vi "Bloomy BS120x Data Logging Example.vi"() -> ()   [LabVIEW 2021]
uses:
  src/TypeDefs/UnitType.ctl
  src/Public/New BS120x Device/New BS120x Ethernet Device.vi
  src/Public/New BS120x Device/New BS120x XNET Device.vi
  src/BS120x.lvclass
  src/BS120x Driver.lvlib
panel:
  in  "Tab Control":enum32{"Basic Control", "Plotting"}(tab)
  out "Protocol":enum32{"CAN", "Ethernet"}(tab)=enum."Ethernet"
  out "Box IDs":u8[](array[numeric])=[1]
  in  "CAN Interface":refnum<k21>
  in  "Current Box ID":u8
  out "Box IP address":string="192.168.1.101"
  out "TCP port":u16=12345
  out "UDP port":u16=54321
  in  "Reset Unit":bool
  in  "Voltage":dbl=5.0 min=0.0 max=5.0 step=0.5
  in  "Source \nCurrent":dbl
  in  "Sink \nCurrent":dbl
  in  "State":bool
  out "Cell Voltages":dbl[](array[numeric])
  out "Cell Current":dbl[](array[numeric]) format="%#8.1f"
  in  "PID Disable":bool
  in  "Precision":bool
  out "Unit Type":T1=enum."BS1201"
  in  "Channel":u16(ring) items=["All", "1", "2", "3", "4", "5", "6", "7", "8", "9", "10", "11", "12"]
  out "error out":errorcluster
  in  "Logging State":enum32{"On", "Off"}(radio)
  in  "Data Log Path":path
  out "Cell Voltages":T2(graph)
  out "Cell Currents":T3(graph)
  in  "Acquisition Rate (Hz)":i32=100 min=1 max=100 step=1
  in  "stop":bool
  # "(c) 2025 Bloomy Controls, Inc. All rights reserved."
  # "Initialization & Configuration"
  # "Cell Control & Readback"
  # "Readback Data"
  # "Control Outputs"
  # "1"
  # "V"
  # "6"
  # "mA"
  # "Operational Config\n(BS1201 Only)"
  # "mA"
  # "12"
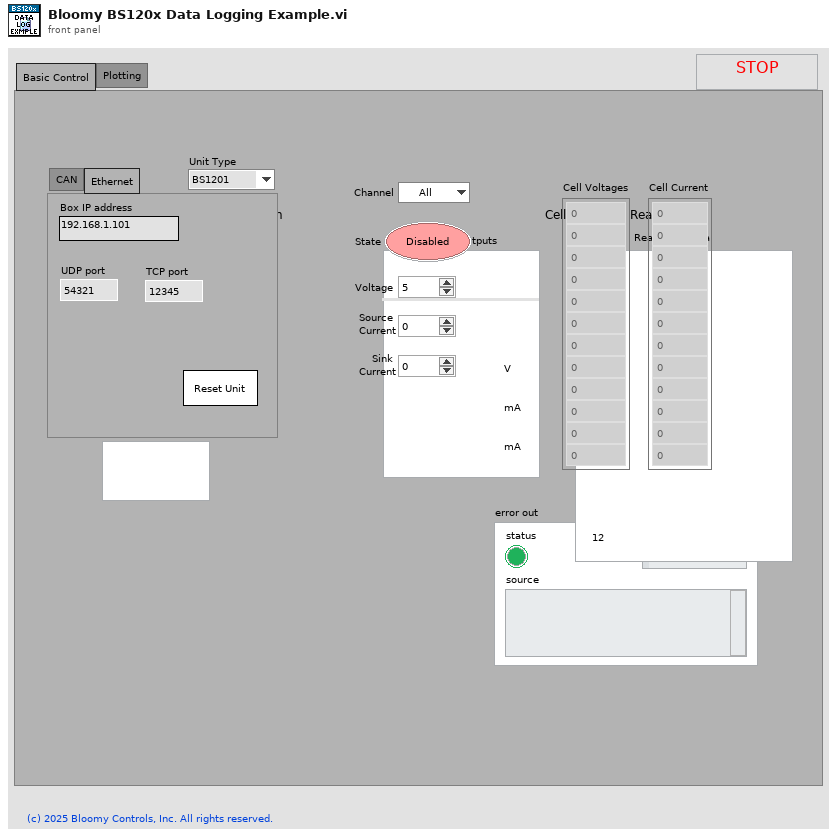
[diagram p1: front panel]
types:
  T1 = typedef "BS120x Driver.lvlib/BS120x.lvclass/UnitType.ctl" = enum16{"BS1200", "BS1201"}
  T2 = cluster{"Voltage[0]":dbl, "Voltage[1]":dbl, "Voltage[2]":dbl, "Voltage[3]":dbl, "Voltage[4]":dbl, "Voltage[5]":dbl, "Voltage[6]":dbl, "Voltage[7]":dbl, "Voltage[8]":dbl, "Voltage[9]":dbl, "Voltage[10]":dbl, "Voltage[11]":dbl}
  T3 = cluster{"Current[0]":dbl, "Current[1]":dbl, "Current[2]":dbl, "Current[3]":dbl, "Current[4]":dbl, "Current[5]":dbl, "Current[6]":dbl, "Current[7]":dbl, "Current[8]":dbl, "Current[9]":dbl, "Current[10]":dbl, "Current[11]":dbl}
  T4 = typedef "BS120x Driver.lvlib/DiscoveredDevice.ctl" = cluster{"Unit Type":T1, "Serial Number":string, "Protocol":T5, "IP Address":string, "UDP Port":u16, "TCP Port":u16, "XNET Box ID":u8, "OS":string, "Firmware Version":string}
  T5 = typedef "BS120x Driver.lvlib/BS120x.lvclass/Protocol.ctl" = enum16{"CAN", "Ethernet"}
  T6 = enum16{"open", "replace", "create", "open or create", "replace or create", "replace or create with confirmation"}
  T7 = cluster{"name (unnamed)":string, "name (unnamed)":string}
  T8 = cluster{"name (unnamed)":string, "NewVal":enum32{"On", "Off"}}
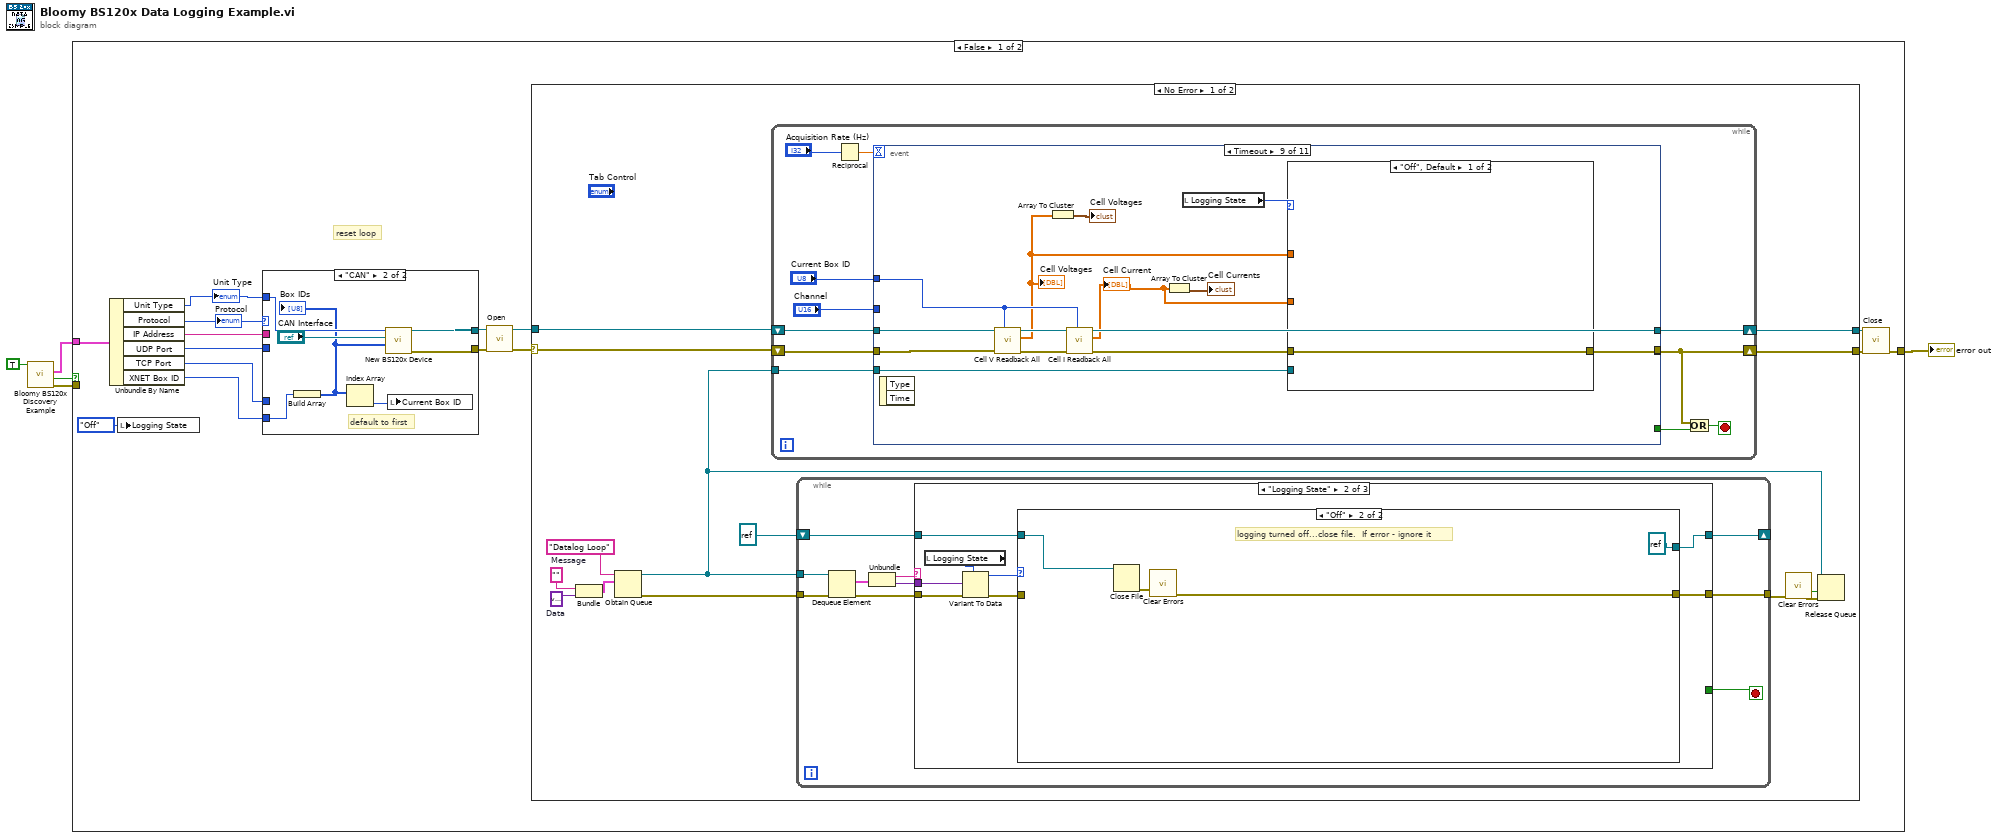
[diagram p0: block diagram]
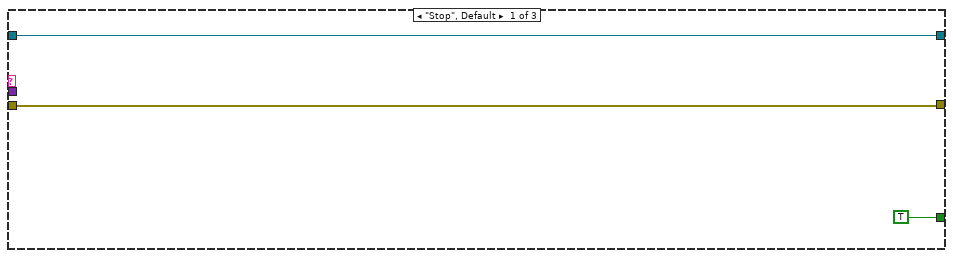
[diagram p2: hidden frame]
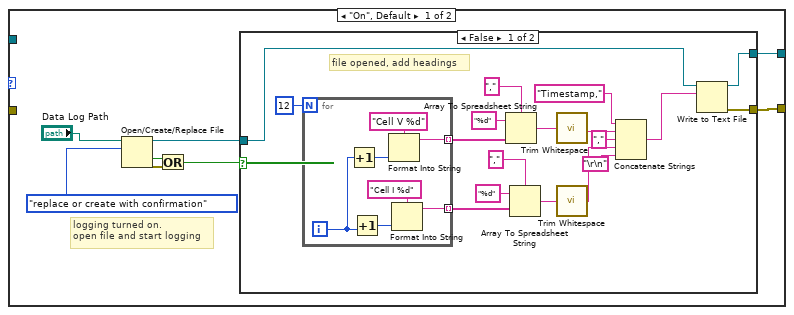
[diagram p3: hidden frame]
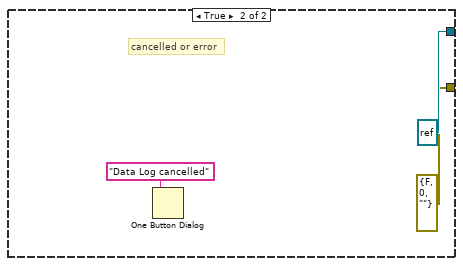
[diagram p4: hidden frame]
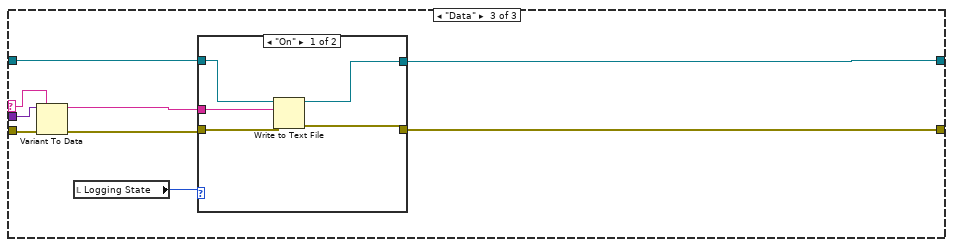
[diagram p5: hidden frame]
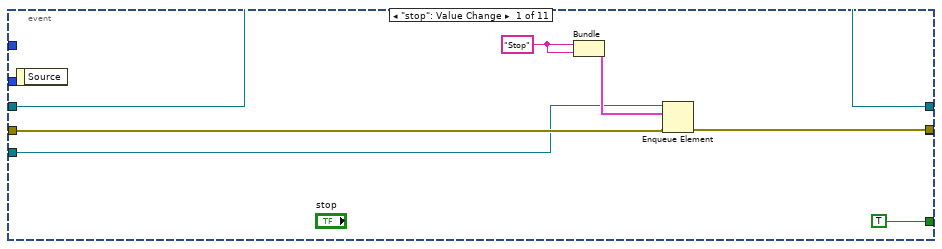
[diagram p7: hidden frame]
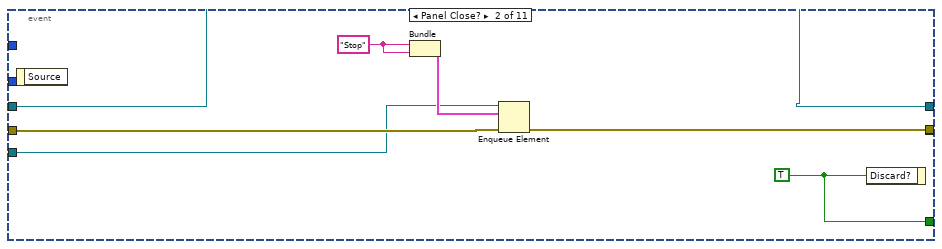
[diagram p8: hidden frame]
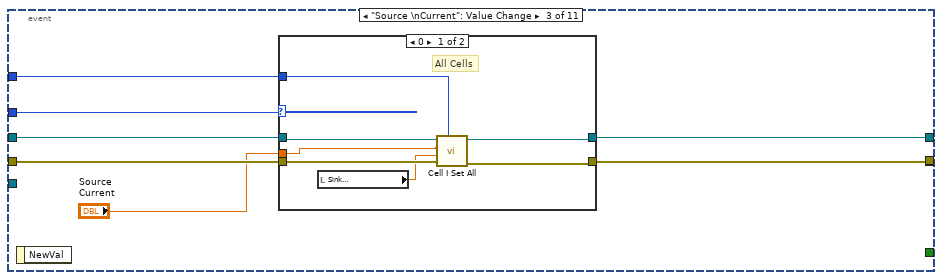
[diagram p9: hidden frame]
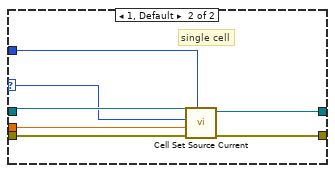
[diagram p10: hidden frame]
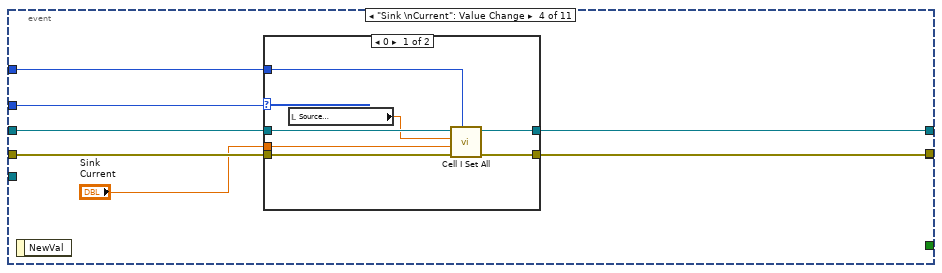
[diagram p11: hidden frame]
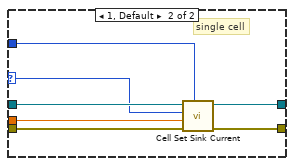
[diagram p12: hidden frame]
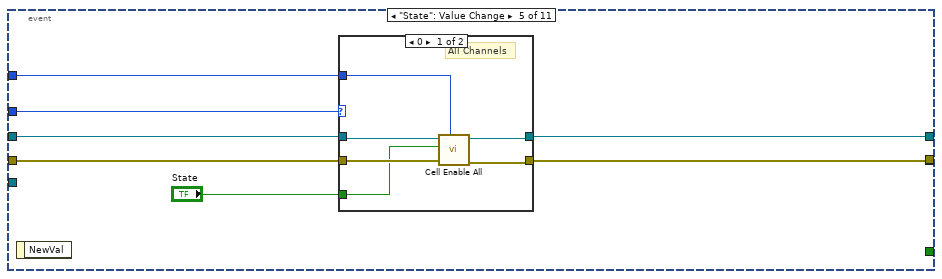
[diagram p13: hidden frame]
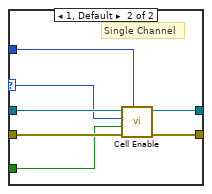
[diagram p14: hidden frame]
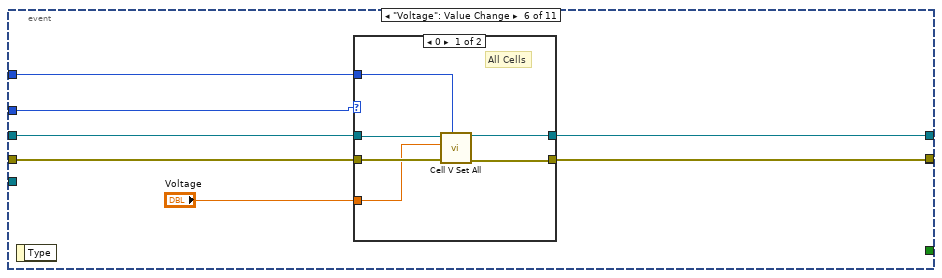
[diagram p15: hidden frame]
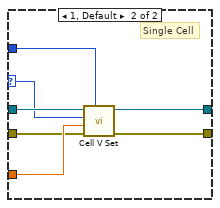
[diagram p16: hidden frame]
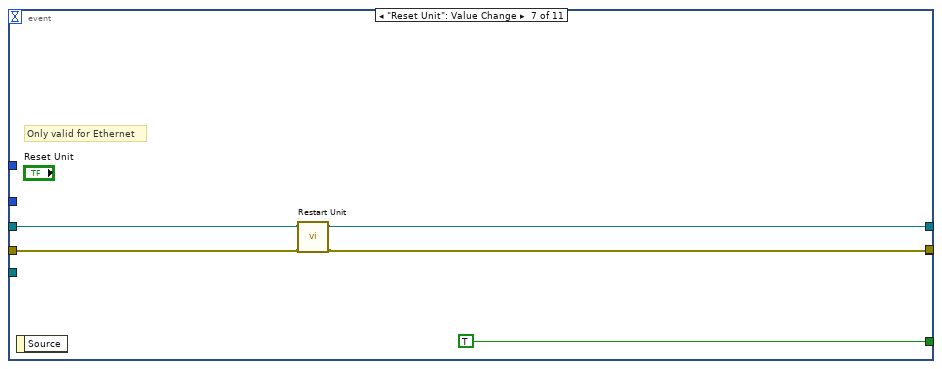
[diagram p17: hidden frame]
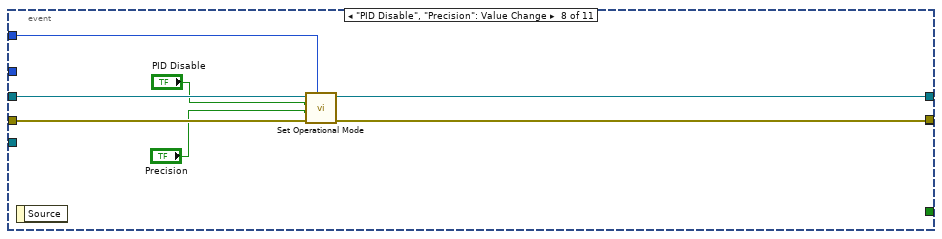
[diagram p18: hidden frame]
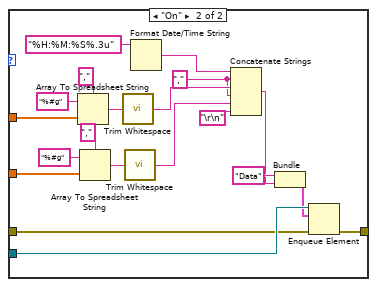
[diagram p19: hidden frame]
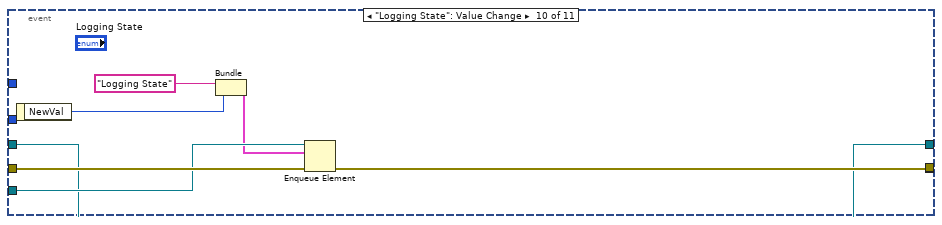
[diagram p20: hidden frame]
diagram:
  n1 = call "Bloomy BS120x Discovery Example.vi"("Allow Selection"=TRUE) -> ("error out"=w2:errorcluster, "Canceled"=w3:bool, "Selected Device"=w1:T4)  [unwired: 7 in, 1 out]
  n2 = case shown="False" w3 {
    tunnel: [w15 w290] -> w5
    tunnel: w2 -> [_ w290]
    tunnel: w1 -> [w13 _]
    frame False {
      # "reset loop"
      n3 = Unbundle By Name(w13) -> ("Unit Type"=w12:T1, "Protocol"=w11:T5, "IP Address"=w10:string, "UDP Port"=w9:u16, "TCP Port"=w8:u16, "XNET Box ID"=w7:u8)
      "Unit Type" <- w12
      "Protocol" <- w11
      n4 = local write "Logging State"(enum32{"On", "Off"}."Off" ("Logging State")) -> ()
      n5 = case shown="\"CAN\"" w11 {
        tunnel: w12 -> [w282 w287]
        tunnel: [w281 w289] -> w18
        tunnel: [w280 w288] -> w16
        tunnel: w10 -> [w279 _]
        tunnel: w9 -> [w278 _]
        tunnel: w8 -> [w277 _]
        tunnel: w7 -> [_ w283]
        frame "Ethernet", Default {
          n6 = call-poly "New BS120x Device.vi"("TCP port"=w277, "UDP port"=w278, "Box IP address"=w279, "Unit Type"=w282) -> ("error out"=w280:errorcluster, "BS120x Out"=w281:refnum<class "BS120x.lvclass">)  [unwired: 6 in]
          "Box IP address" <- w279
          "TCP port" <- w277
          "UDP port" <- w278
        }
        frame "CAN" {
          # "default to first"
          n7 = Build Array(w283) -> (w284:u8[])
          "Box IDs" <- w284
          n8 = Index Array(array=w284) -> (element=w285:u8)  [unwired: 1 in]
          n9 = call-poly "New BS120x Device.vi"("Box IDs"=w284, "CAN Interface"="CAN Interface", "Unit Type"=w287) -> ("error out"=w288:errorcluster, "BS120x out"=w289:refnum<class "BS120x.lvclass">)  [unwired: 7 in]
          n10 = local write "Current Box ID"(w285) -> ()
        }
      }
      n11 = call-dynamic "Open.vi"("error in (no error)"=w16, "BS120x in"=w18) -> ("error out"=w14:errorcluster, "BS120x out"=w17:refnum<class "BS120x.lvclass">)  [unwired: 8 in]
      n12 = case shown="No Error" w14 {
        selector: w14 -> [w31 w275]
        tunnel: [w34 w275] -> w20
        tunnel: [w33 w276] -> w19
        tunnel: w17 -> [w32 w276]
        frame No Error {
          w27 = variant  # Data
          w28 = ""  # Message
          n13 = Bundle("Message"=w28, "Data"=w27) -> (w26:cluster{"Message":string, "Data":variant})  [unwired: 1 in]
          n14 = Obtain Queue(name (unnamed)="Datalog Loop", element data type=w26) -> (queue out=w21:refnum<queue>, error out=w25:errorcluster)  [unwired: 3 in, 1 out]
          n15 = while {
            shift-right: [w117] -> w34
            shift-left: w31 -> [w120]
            shift-right: [w122] -> w33
            shift-left: w32 -> [w121]
            tunnel: w21 -> [w112]
            stop <- w119 stop-if-true
            n16 = Reciprocal(x="Acquisition Rate (Hz)") -> (1/x=w113:dbl)
            n17 = event shown="[8] Timeout" {
              selector: _ -> [_ _ _ _ _ _ _ _ _ _ _]
              dyn-events: _ -> [_ _ _ _ _ _ _ _ _ _ _]
              timeout: w113 -> [_ _ _ _ _ _ _ _ _ _ _]
              tunnel: [w128 w133 w140 w161 w183 w201 w220 w227 w244 w267 w274] -> w122
              tunnel: w121 -> [w128 w133 w143 w164 w184 w204 w219 w228 w232 w267 w274]
              tunnel: [w126 _ w141 w160 w182 w202 w221 w229 w239 w268 w273] -> w117
              tunnel: w120 -> [w127 w132 w142 w163 w185 w203 w222 w230 w231 w272 w273]
              tunnel: [TRUE ("Discard?") w136 _ _ _ _ TRUE ("Discard?") _ _ _ _] -> w118
              tunnel: "Channel" -> [_ _ w138 w159 w180 w200 _ _ _ _ _]
              tunnel: "Current Box ID" -> [_ _ w137 w158 w179 w199 _ w224 w241 _ _]
              tunnel: w112 -> [w125 w130 _ _ _ _ _ _ w233 w271 _]
              tunnel: [_ w131 _ _ _ _ _ _ _ _ _] -> _
              event "stop": Value Change {
                w124 = "Stop" ("name (unnamed)")
                n18 = event-data() -> ()  [unwired: 1 in, 1 out]
                n19 = Bundle("name (unnamed)"=w124, "name (unnamed)"=w124) -> (w129:T7)  [unwired: 1 in]
                n20 = Enqueue Element(queue=w125, element=w129, error in (no error)=w127) -> (error out=w126:errorcluster)  [unwired: 1 in, 2 out]
              }
              event Panel Close? {
                w134 = "Stop" ("name (unnamed)")
                w136 = TRUE ("Discard?")
                n21 = event-data() -> ()  [unwired: 1 in, 1 out]
                n22 = Bundle("name (unnamed)"=w134, "name (unnamed)"=w134) -> (w135:T7)  [unwired: 1 in]
                n23 = Enqueue Element(queue=w130, element=w135, error in (no error)=w132) -> (error out=w131:errorcluster)  [unwired: 1 in, 2 out]
                n24 = event-data("Discard?"=w136) -> ()  [unwired: 1 in, 1 out]
              }
              event "Source \nCurrent": Value Change {
                n25 = event-data() -> ()  [unwired: 1 in, 1 out]
                n26 = case shown="0" w138 {
                  selector: w138 -> [_ w152]
                  tunnel: w143 -> [w149 w157]
                  tunnel: w142 -> [w148 w156]
                  tunnel: [w147 w155] -> w141
                  tunnel: [w150 w154] -> w140
                  tunnel: "Source \nCurrent" -> [w146 w153]
                  tunnel: w137 -> [w144 w151]
                  frame 0 {
                    # "All Cells"
                    n27 = local read "Sink \nCurrent"() -> (w145:dbl)
                    n28 = call-dynamic "Cell I Set All.vi"("Box ID"=w144, "error in (no error)"=w148, "Sink I All"=w145, "Source I All"=w146, "BS120x in"=w149) -> ("error out"=w147:errorcluster, "BS120x out"=w150:refnum<class "BS120x.lvclass">)  [unwired: 5 in]
                  }
                  frame 1, Default {
                    # "single cell"
                    n29 = call-dynamic "Cell Set Source Current.vi"("Box ID"=w151, "error in (no error)"=w156, "Source Current Limit (mA)"=w153, "Channel"=w152, "BS120x in"=w157) -> ("error out"=w155:errorcluster, "BS120x out"=w154:refnum<class "BS120x.lvclass">)  [unwired: 5 in]
                  }
                }
              }
              event "Sink \nCurrent": Value Change {
                n30 = event-data() -> ()  [unwired: 1 in, 1 out]
                n31 = case shown="0" w159 {
                  selector: w159 -> [_ w173]
                  tunnel: w164 -> [w169 w178]
                  tunnel: w163 -> [w168 w177]
                  tunnel: "Sink \nCurrent" -> [w167 w176]
                  tunnel: [w170 w175] -> w161
                  tunnel: [w171 w174] -> w160
                  tunnel: w158 -> [w165 w172]
                  frame 0 {
                    n32 = local read "Source \nCurrent"() -> (w166:dbl)
                    n33 = call-dynamic "Cell I Set All.vi"("Box ID"=w165, "error in (no error)"=w168, "Sink I All"=w167, "Source I All"=w166, "BS120x in"=w169) -> ("error out"=w171:errorcluster, "BS120x out"=w170:refnum<class "BS120x.lvclass">)  [unwired: 5 in]
                  }
                  frame 1, Default {
                    # "single cell"
                    n34 = call-dynamic "Cell Set Sink Current.vi"("Box ID"=w172, "error in (no error)"=w177, "Sink Current Limit (mA)"=w176, "Channel"=w173, "BS120x in"=w178) -> ("error out"=w174:errorcluster, "BS120x out"=w175:refnum<class "BS120x.lvclass">)  [unwired: 5 in]
                  }
                }
              }
              event "State": Value Change {
                n35 = event-data() -> ()  [unwired: 1 in, 1 out]
                n36 = case shown="0" w180 {
                  selector: w180 -> [_ w193]
                  tunnel: w185 -> [w190 w198]
                  tunnel: w184 -> [w191 w197]
                  tunnel: [w189 w196] -> w183
                  tunnel: [w188 w195] -> w182
                  tunnel: "State" -> [w187 w194]
                  tunnel: w179 -> [w186 w192]
                  frame 0 {
                    # "All Channels"
                    n37 = call-dynamic "Cell Enable All.vi"("Box ID"=w186, "error in (no error)"=w190, "Enable"=w187, "BS120x in"=w191) -> ("error out"=w188:errorcluster, "BS120x out"=w189:refnum<class "BS120x.lvclass">)  [unwired: 6 in]
                  }
                  frame 1, Default {
                    # "Single Channel"
                    n38 = call-dynamic "Cell Enable.vi"("Box ID"=w192, "error in (no error)"=w198, "Enable"=w194, "Channel"=w193, "BS120x in"=w197) -> ("error out"=w195:errorcluster, "BS120x out"=w196:refnum<class "BS120x.lvclass">)  [unwired: 5 in]
                  }
                }
              }
              event "Voltage": Value Change {
                n39 = event-data() -> ()  [unwired: 1 in, 1 out]
                n40 = case shown="0" w200 {
                  selector: w200 -> [_ w213]
                  tunnel: "Voltage" -> [w207 w218]
                  tunnel: w204 -> [w211 w217]
                  tunnel: w203 -> [w210 w216]
                  tunnel: [w209 w215] -> w202
                  tunnel: [w208 w214] -> w201
                  tunnel: w199 -> [w206 w212]
                  frame 0 {
                    # "All Cells"
                    n41 = call-dynamic "Cell V Set All.vi"("Box ID"=w206, "error in (no error)"=w210, "Voltage"=w207, "BS120x in"=w211) -> ("error out"=w209:errorcluster, "BS120x out"=w208:refnum<class "BS120x.lvclass">)  [unwired: 6 in]
                  }
                  frame 1, Default {
                    # "Single Cell"
                    n42 = call-dynamic "Cell V Set.vi"("Box ID"=w212, "error in (no error)"=w216, "Voltage"=w218, "Channel"=w213, "BS120x in"=w217) -> ("error out"=w215:errorcluster, "BS120x out"=w214:refnum<class "BS120x.lvclass">)  [unwired: 5 in]
                  }
                }
              }
              event "Reset Unit": Value Change {
                # "Only valid for Ethernet"
                n43 = event-data() -> ()  [unwired: 1 in, 1 out]
                n44 = call-dynamic "Restart Unit.vi"("error in (no error)"=w222, "BS120x in"=w219) -> ("error out"=w221:errorcluster, "BS120x out"=w220:refnum<class "BS120x.lvclass">)  [unwired: 8 in]
              }
              event "PID Disable", "Precision": Value Change {
                n45 = event-data() -> ()  [unwired: 1 in, 1 out]
                n46 = call-dynamic "Set Operational Mode.vi"("Box ID"=w224, "error in (no error)"=w230, "Precision Mode"="Precision", "PID Disable"="PID Disable", "BS120x in"=w228) -> ("error out"=w229:errorcluster, "BS120x out"=w227:refnum<class "BS120x.lvclass">)  [unwired: 5 in]
              }
              event Timeout {
                n47 = event-data() -> ()  [unwired: 1 in, 2 out]
                n48 = call-dynamic "Cell V Readback All.vi"("Box ID"=w241, "error in (no error)"=w231, "BS120x in"=w232) -> ("error out"=w242:errorcluster, "Voltage"=w234:dbl[], "BS120x out"=w243:refnum<class "BS120x.lvclass">)  [unwired: 6 in]
                "Cell Voltages" <- w234
                n49 = Array To Cluster(array=w234) -> (cluster=→"Cell Voltages":T2)
                n50 = call-dynamic "Cell I Readback All.vi"("Box ID"=w241, "error in (no error)"=w242, "BS120x in"=w243) -> ("error out"=w240:errorcluster, "Current"=w235:dbl[], "BS120x out"=w244:refnum<class "BS120x.lvclass">)  [unwired: 6 in]
                "Cell Current" <- w235
                n51 = Array To Cluster(array=w235) -> (cluster=→"Cell Currents":T3)
                n52 = local read "Logging State"() -> (w238:enum32{"On", "Off"})
                n53 = case shown="\"Off\", Default" w238 {
                  tunnel: w234 -> [_ w265]
                  tunnel: w235 -> [_ w258]
                  tunnel: w240 -> [w245 w246]
                  tunnel: [w245 w251] -> w239
                  tunnel: w233 -> [_ w250]
                  frame "Off", Default {
                  }
                  frame "On" {
                    w252 = "," ("string")
                    n54 = Array To Spreadsheet String(delimiter (Tab)=",", array=w265, 3:"%#g" ("format string")) -> (spreadsheet string=w262:string)
                    n55 = Array To Spreadsheet String(delimiter (Tab)=",", array=w258, 3:"%#g" ("format string")) -> (spreadsheet string=w261:string)
                    n56 = call <vilib>:"Trim Whitespace.vi"("string"=w262) -> ("trimmed string"=w257:string)  [unwired: 1 in]
                    n57 = call <vilib>:"Trim Whitespace.vi"("string"=w261) -> ("trimmed string"=w256:string)  [unwired: 1 in]
                    n58 = Format Date/Time String(time format string (%c)="%H:%M:%S%.3u") -> (date/time string=w253:string)  [unwired: 2 in]
                    n59 = Concatenate Strings(w253, w252, w257, w252, w256, "\r\n") -> (w248:string)
                    n60 = Bundle("name (unnamed)"="Data", w248) -> (w247:cluster{"name (unnamed)":string, string})  [unwired: 1 in]
                    n61 = Enqueue Element(queue=w250, element=w247, error in (no error)=w246) -> (error out=w251:errorcluster)  [unwired: 1 in, 2 out]
                  }
                }
              }
              event "Logging State": Value Change {
                n62 = event-data() -> ("NewVal"=w266:enum32{"On", "Off"})  [unwired: 1 in]
                n63 = Bundle("name (unnamed)"="Logging State", "NewVal"=w266) -> (w269:T8)  [unwired: 1 in]
                n64 = Enqueue Element(queue=w271, element=w269, error in (no error)=w272) -> (error out=w268:errorcluster)  [unwired: 1 in, 2 out]
              }
              event "Channel": Value Change {
                # "force changes to this control to be read by resetting the loop"
                n65 = event-data() -> ()  [unwired: 1 in, 4 out]
              }
            }
            n66 = Or(x=w117, y=w118) -> (x .or. y?=w119:bool)
          }
          n67 = while {
            shift-right: [w37] -> _
            shift-left: refnum<file> refnum ("refnum out") -> [w38]
            tunnel: w21 -> [w44]
            tunnel: w25 -> [w43]
            tunnel: [w36] -> w22
            stop <- w35 stop-if-true
            n68 = Dequeue Element(queue=w44, error in (no error)=w43) -> (element=w42:cluster{"Message":string, "Data":variant}, error out=w40:errorcluster)  [unwired: 1 in, 2 out]
            n69 = Unbundle(w42) -> ("Message"=w41:string, "Data"=w39:variant)
            n70 = case shown="\"Logging State\"" w41 {
              selector: w41 -> [_ _ w102]
              tunnel: w40 -> [w45 w53 w104]
              tunnel: w39 -> [_ w52 w103]
              tunnel: w38 -> [w47 w48 w100]
              tunnel: [w47 w55 w99] -> w37
              tunnel: [w45 w54 w96] -> w36
              tunnel: [TRUE _ _] -> w35
              frame "Stop", Default {
              }
              frame "Logging State" {
                n71 = local read "Logging State"() -> (w51:enum32{"On", "Off"})
                n72 = Variant To Data(error in=w53, type=w51, Variant=w52) -> (data=w50:enum32{"On", "Off"}, error out=w49:errorcluster)
                n73 = case shown="\"Off\"" w50 {
                  tunnel: [w59 refnum<file> refnum ("refnum out")] -> w55
                  tunnel: [w57 w94] -> w54
                  tunnel: w49 -> [_ _]
                  tunnel: w48 -> [_ w92]
                  frame "On", Default {
                    # "logging turned on.  \nopen file and start logging"
                    n74 = Open/Create/Replace File(file path (use dialog)="Data Log Path", operation (0:open)=T6."replace or create with confirmation") -> (refnum out=w58:refnum<file>, cancelled=w62:bool, error out=w61:errorcluster)  [unwired: 4 in]
                    n75 = Or(x=w62, y=w61) -> (x .or. y?=w60:bool)
                    n76 = case shown="False" w60 {
                      tunnel: [w81 refnum<file> refnum ("refnum out")] -> w59
                      tunnel: w58 -> [w66 _]
                      tunnel: [w80 errorcluster {"status"=FALSE, "code"=0, "source"=""} ("error out")] -> w57
                      frame False {
                        # "file opened, add headings"
                        n77 = for {
                          N: 12 -> [_]
                          tunnel: [w83] -> w74 mode=indexing
                          tunnel: [w82] -> w75 mode=indexing
                          i -> [w86]
                          n78 = Increment(x=w86) -> (x+1=w88:i32)
                          n79 = Increment(x=w86) -> (x+1=w87:i32)
                          n80 = Format Into String(format string="Cell V %d", w88) -> (resulting string=w83:string)  [unwired: 2 in, 1 out]
                          n81 = Format Into String(format string="Cell I %d", w87) -> (resulting string=w82:string)  [unwired: 2 in, 1 out]
                        }
                        n82 = Array To Spreadsheet String(delimiter (Tab)=",", array=w74, 3:"%d" ("format string")) -> (spreadsheet string=w76:string)
                        n83 = Array To Spreadsheet String(delimiter (Tab)=",", array=w75, 3:"%d" ("format string")) -> (spreadsheet string=w77:string)
                        n84 = call <vilib>:"Trim Whitespace.vi"("string"=w76) -> ("trimmed string"=w79:string)  [unwired: 1 in]
                        n85 = call <vilib>:"Trim Whitespace.vi"("string"=w77) -> ("trimmed string"=w78:string)  [unwired: 1 in]
                        n86 = Concatenate Strings("Timestamp," ("text"), w79, "," ("string"), w78, "\r\n") -> (w65:string)
                        n87 = Write to Text File(file (use dialog)=w66, text=w65) -> (refnum out=w81:refnum<file>, error out=w80:errorcluster)  [unwired: 2 in, 1 out]
                      }
                      frame True {
                        # "cancelled or error"
                        n88 = One Button Dialog(message="Data Log cancelled") -> ()  [unwired: 1 in, 1 out]
                      }
                    }
                  }
                  frame "Off" {
                    # "logging turned off...close file.  If error - ignore it"
                    n89 = Close File(refnum=w92) -> (error out=w95:errorcluster)  [unwired: 1 in, 1 out]
                    n90 = call <vilib>:"Clear Errors.vi"("error in (no error)"=w95) -> ("error out"=w94:errorcluster)  [unwired: 5 in, 1 out]
                  }
                }
              }
              frame "Data" {
                n91 = Variant To Data(error in=w104, type=w102, Variant=w103) -> (data=w97:string, error out=w98:errorcluster)
                n92 = local read "Logging State"() -> (w101:enum32{"On", "Off"})
                n93 = case shown="\"On\"" w101 {
                  tunnel: w100 -> [w109 w111]
                  tunnel: [w108 w111] -> w99
                  tunnel: [w106 w110] -> w96
                  tunnel: w98 -> [w107 w110]
                  tunnel: w97 -> [w105 _]
                  frame "On" {
                    n94 = Write to Text File(file (use dialog)=w109, text=w105, error in=w107) -> (refnum out=w108:refnum<file>, error out=w106:errorcluster)  [unwired: 1 in, 1 out]
                  }
                  frame "Off", Default {
                  }
                }
              }
            }
          }
          n95 = call <vilib>:"Clear Errors.vi"("error in (no error)"=w22) -> ("error out"=w24:errorcluster, "specific error cleared?"=w23:bool)  [unwired: 5 in]
          n96 = Release Queue(queue=w21, force destroy? (F)=w23, error in (no error)=w24) -> ()  [unwired: 3 out]
        }
        frame Error {
        }
      }
      n97 = call-dynamic "Close.vi"("error in (no error)"=w20, "BS120x In"=w19) -> ("error out"=w15:errorcluster)  [unwired: 8 in, 1 out]
    }
    frame True {
    }
  }
  "error out" <- w5
